vi "Create Queue CMain.vi"(8 "error in":errorcluster) -> (0 "error out":errorcluster, 3 "queCMain":refnum<queue>)   [LabVIEW 2016]
uses:
  Library/Event/Ctl/EventVariantData.ctl
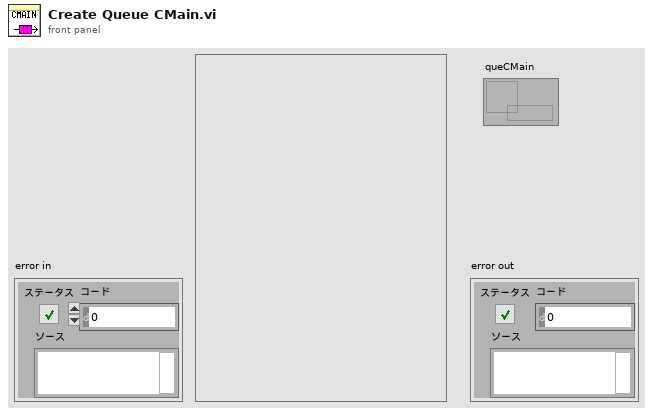
[diagram p1: front panel]
types:
  T1 = typedef "EventVariantData.ctl" = cluster{"コマンド":string, "バリアント":variant}
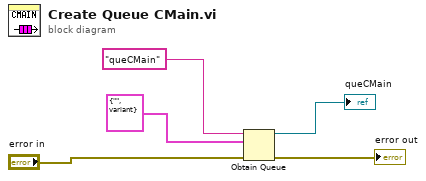
[diagram p0: block diagram]
diagram:
  n1 = Obtain Queue(name (unnamed)="queCMain" ("名前（名前なし）"), element data type=T1 {"コマンド"="", "バリアント"=variant}, error in (no error)="error in") -> (queue out=→"queCMain":refnum<queue>, error out=→"error out":errorcluster)  [unwired: 2 in, 1 out]
